vi "AIT 1553 - Write FIFOs.vi"(5 "Bus Section":T1, 7 "Mode":T2, 8 "error in (no error)":errorcluster, 11 "RT Data in":T3 {"Acyclic Frame Refs" format="%.0x"; "Label Transfer Config"."Block Data Refs"."Data Reference" format="%.0x"; "Status Config"."HWOut Dur Ref" format="%.0x"; "Status Config"."HWIn Dur Ref" format="%.0x"; "Status Config"."HWOut Count Ref" format="%.0x"; "Status Config"."HWIn Count Ref" format="%.0x"; "Status Config"."Error Data Ref" format="%.0x"; "HWOutput Channels"."Message Settings"."Driver Data"."First Word" min=8 max=31; "HWOutput Channels"."Message Settings"."Driver Data"."Num Bits" min=1 max=32; "HWOutput Channels"."Message Settings"."Driver Data"."Start Bit" min=8 max=31; "HWOutput Channels"."Message Settings"."Block Data Refs"."Data Reference" format="%.0x"; "HWInput Channels"."Message Settings"."Driver Data"."First Word" min=8 max=31; "HWInput Channels"."Message Settings"."Driver Data"."Num Bits" min=1 max=32; "HWInput Channels"."Message Settings"."Driver Data"."Start Bit" min=8 max=31; "HWInput Channels"."Message Settings"."Block Data Refs"."Data Reference" format="%.0x"}) -> (0 "error out":errorcluster, 3 "RT Data out":T3 {"Acyclic Frame Refs" format="%.0x"; "Label Transfer Config"."Block Data Refs"."Data Reference" format="%.0x"; "Status Config"."HWOut Dur Ref" format="%.0x"; "Status Config"."HWIn Dur Ref" format="%.0x"; "Status Config"."HWOut Count Ref" format="%.0x"; "Status Config"."HWIn Count Ref" format="%.0x"; "Status Config"."Error Data Ref" format="%.0x"; "HWOutput Channels"."Message Settings"."Driver Data"."First Word" min=8 max=31; "HWOutput Channels"."Message Settings"."Driver Data"."Num Bits" min=1 max=32; "HWOutput Channels"."Message Settings"."Driver Data"."Start Bit" min=8 max=31; "HWOutput Channels"."Message Settings"."Block Data Refs"."Data Reference" format="%.0x"; "HWInput Channels"."Message Settings"."Driver Data"."First Word" min=8 max=31; "HWInput Channels"."Message Settings"."Driver Data"."Num Bits" min=1 max=32; "HWInput Channels"."Message Settings"."Driver Data"."Start Bit" min=8 max=31; "HWInput Channels"."Message Settings"."Block Data Refs"."Data Reference" format="%.0x"})   [LabVIEW 2013, in "AIT 1553 Custom Device.lvlib"]
uses:
  AIT 1553 Custom Device.lvlib
  RT Controls/AIT 1553  - RT Data.ctl
  RT Controls/AIT 1553 - RT HW Channel.ctl
  RT Controls/AIT 1553 - Bus Section.ctl
  RT Controls/AIT 1553 - RT Message Settings.ctl
  <vilib>/NI Veristand/Custom Device API/Block Data Reference.ctl
  <vilib>/NI Veristand/Custom Device API/Data Reference.ctl
  RT Controls/AIT 1553 - Driver Data.ctl
  Controls and Global/Start Bit.ctl
  Controls and Global/Number of Bits.ctl
  RT Controls/AIT 1553 - Board Config Info.ctl
  RT Controls/AIT 1553 - Hardware Type.ctl
  RT Controls/Error Qs.ctl
  RT Controls/Status Channels Config.ctl
  RT Controls/FIFO.ctl
  RT Controls/Label Transfer Config.ctl
  <vilib>/NI Veristand/Custom Device API/Custom Device Item Ref.ctl
  RT Controls/ReadWrite Selector.ctl
  <vilib>/NI Veristand/Custom Device API/Custom Device API.lvlib
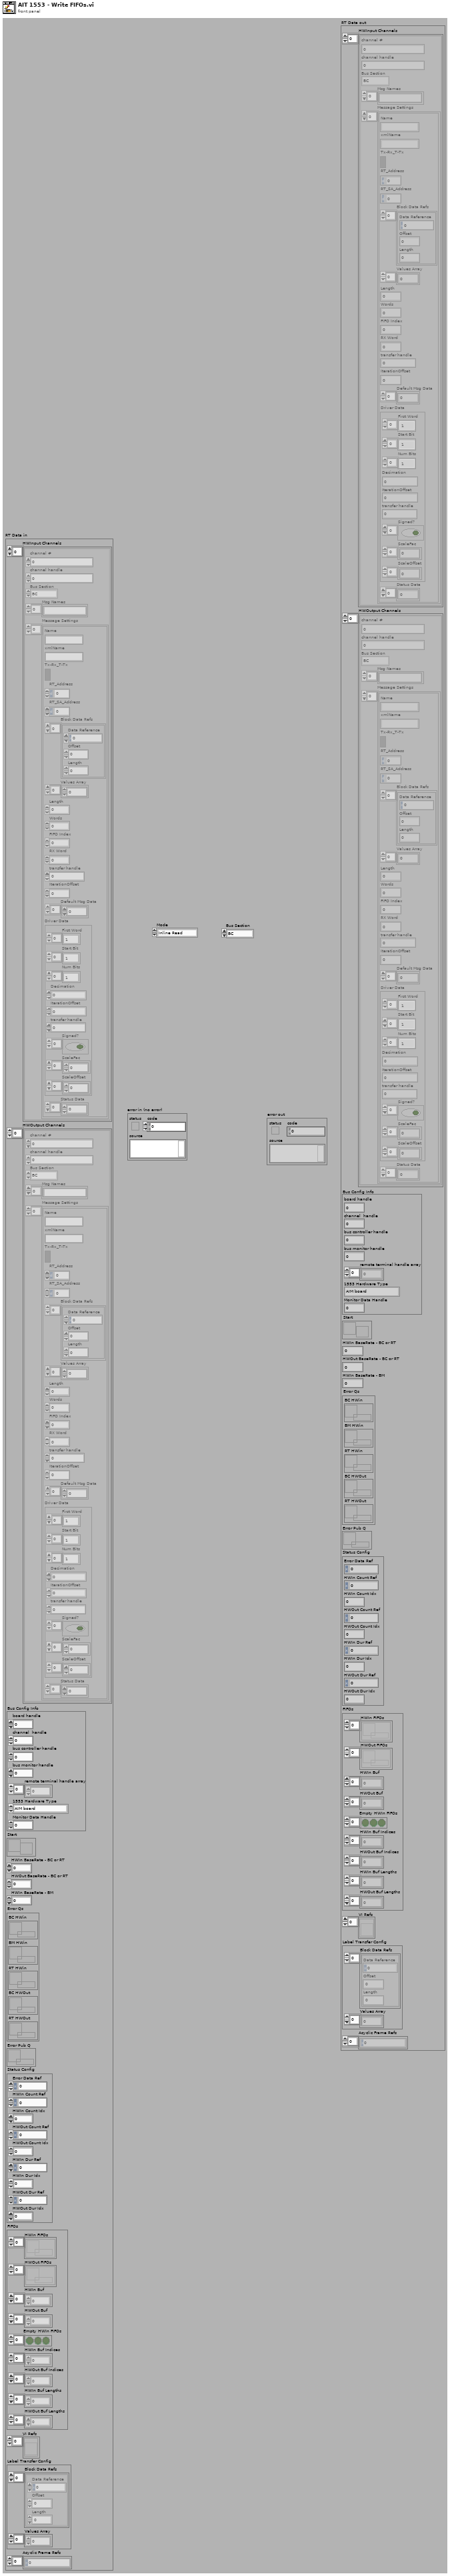
[diagram p1: front panel]
types:
  T1 = typedef "AIT 1553 Custom Device.lvlib/AIT 1553 - Bus Section.ctl" = enum16{"BC", "BM", "RT"}
  T2 = typedef "AIT 1553 Custom Device.lvlib/ReadWrite Selector.ctl" = enum16{"Inline Read", "Inline Write", "Async HWIn", "Async HWOut"}
  T3 = typedef "AIT 1553 Custom Device.lvlib/AIT 1553  - RT Data.ctl" = cluster{"HWInput Channels":T4[], "HWOutput Channels":T4[], "Bus Config Info":T11, "Start":refnum<notifier>, "HWIn BaseRate - BC or RT":i64, "HWOut BaseRate - BC or RT":i64, "HWIn BaseRate - BM":i64, "Error Qs":T13, "Error Pub Q":refnum<queue>, "Status Config":T14, "FIFOs":T15, "VI Refs":refnum<vi>[], "Label Transfer Config":T16, "Acyclic Frame Refs":T17[]}
  T4 = typedef "AIT 1553 Custom Device.lvlib/AIT 1553 - RT HW Channel.ctl" = cluster{"channel #":u16, "channel handle":u32, "Bus Section":T1, "Msg Names":string[], "Message Settings":T5[]}
  T5 = typedef "AIT 1553 Custom Device.lvlib/AIT 1553 - RT Message Settings.ctl" = cluster{"Name":string, "xmlName":string, "Tx-Rx_T-Tx":bool, "RT_Address":u8, "RT_SA_Address":u8, "Block Data Refs":T6[], "Values Array":dbl[], "Length":i32, "Words":i32, "FIFO Index":i32, "RX Word":u32, "transfer handle":u32, "IterationOffset":i32, "Default Msg Data":u16[], "Driver Data":T8, "Status Data":u32[]}
  T6 = typedef "Custom Device API.lvlib/Block Data Reference.ctl" = cluster{"Data Reference":T7, "Offset":i32, "Length":i32}
  T7 = typedef "Custom Device API.lvlib/Data Reference.ctl" = i32
  T8 = typedef "AIT 1553 Custom Device.lvlib/AIT 1553 - Driver Data.ctl" = cluster{"First Word":T9[], "Start Bit":T9[], "Num Bits":T10[], "Decimation":i32, "IterationOffset":i32, "transfer handle":u32, "Signed?":bool[], "ScaleFac":dbl[], "ScaleOffset":dbl[]}
  T9 = typedef "AIT 1553 Custom Device.lvlib/Start Bit.ctl" = i32
  T10 = typedef "AIT 1553 Custom Device.lvlib/Number of Bits.ctl" = i32
  T11 = typedef "AIT 1553 Custom Device.lvlib/AIT 1553 - Board Config Info.ctl" = cluster{"board handle":u32, "channel  handle":u32, "bus controller handle":u32, "bus monitor handle":u32, "remote terminal handle array":u32[], "1553 Hardware Type":T12, "Monitor Data Handle":u32}
  T12 = typedef "AIT 1553 Custom Device.lvlib/AIT 1553 - Hardware Type.ctl" = enum16{"AIM board", "AIT Board"}
  T13 = typedef "AIT 1553 Custom Device.lvlib/Error Qs.ctl" = cluster{"BC HWin":refnum<queue>, "BM HWin":refnum<queue>, "RT HWin":refnum<queue>, "BC HWOut":refnum<queue>, "RT HWOut":refnum<queue>}
  T14 = typedef "AIT 1553 Custom Device.lvlib/Status Channels Config.ctl" = cluster{"Error Data Ref":T7, "HWIn Count Ref":T7, "HWIn Count Idx":i32, "HWOut Count Ref":T7, "HWOut Count Idx":i32, "HWIn Dur Ref":T7, "HWIn Dur Idx":i32, "HWOut Dur Ref":T7, "HWOut Dur Idx":i32}
  T15 = typedef "AIT 1553 Custom Device.lvlib/FIFO.ctl" = cluster{"HWIn FIFOs":refnum<k33>[], "HWOut FIFOs":refnum<k33>[], "HWIn Buf":dbl[], "HWOut Buf":dbl[], "Empty HWIn FIFOs":bool[], "HWIn Buf Indices":i32[], "HWOut Buf Indices":i32[], "HWIn Buf Lengths":i32[], "HWOut Buf Lengths":i32[]}
  T16 = typedef "AIT 1553 Custom Device.lvlib/Label Transfer Config.ctl" = cluster{"Block Data Refs":T6[], "Values Array":dbl[]}
  T17 = typedef "Custom Device API.lvlib/Custom Device Item Ref.ctl" = u64
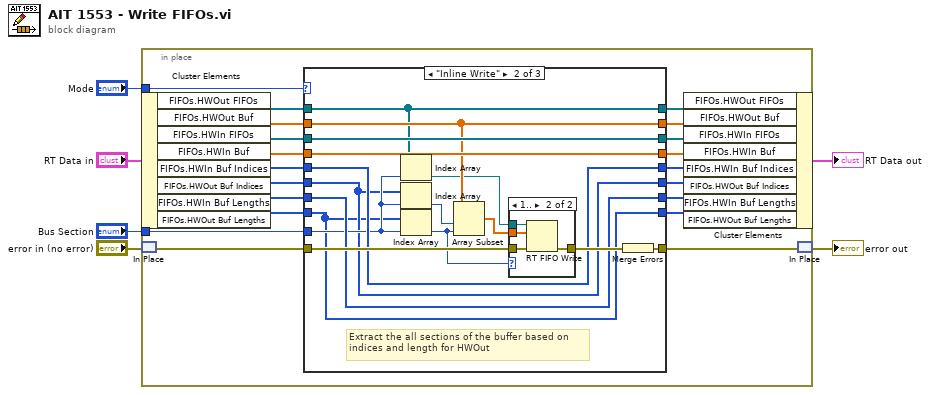
[diagram p0: block diagram]
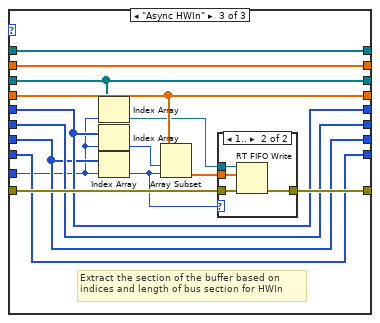
[diagram p4: hidden frame]
diagram:
  n1 = in-place {
    in-place-border: "Mode" -> [w20]
    in-place-border: "Bus Section" -> [w7]
    n2 = in-place-cluster #1("RT Data in") -> ("FIFOs.HWOut FIFOs"=w19:refnum<k33>[], "FIFOs.HWOut Buf"=w18:dbl[], "FIFOs.HWIn FIFOs"=w26:refnum<k33>[], "FIFOs.HWIn Buf"=w25:dbl[], "FIFOs.HWIn Buf Indices"=w15:i32[], "FIFOs.HWOut Buf Indices"=w14:i32[], "FIFOs.HWIn Buf Lengths"=w13:i32[], "FIFOs.HWOut Buf Lengths"=w12:i32[])
    n3 = in-place-match #2("error in (no error)") -> (w22:errorcluster)
    n4 = case shown="\"Inline Write\"" w20 {
      tunnel: w26 -> [w34 w49 w60]
      tunnel: w25 -> [w35 w50 w65]
      tunnel: [w35 w50 w65] -> w24
      tunnel: [w34 w49 w60] -> w23
      tunnel: w22 -> [w33 w51 w69]
      tunnel: [w33 w46 w68] -> w21
      tunnel: w19 -> [w31 w45 w71]
      tunnel: w18 -> [w32 w47 w70]
      tunnel: [w31 w45 w71] -> w17
      tunnel: [w32 w47 w70] -> w16
      tunnel: [w30 w43 w63] -> w11
      tunnel: w15 -> [w30 w43 w63]
      tunnel: [w29 w37 w66] -> w10
      tunnel: w14 -> [w29 w37 w66]
      tunnel: [w28 w42 w62] -> w9
      tunnel: w13 -> [w28 w42 w62]
      tunnel: [w27 w36 w67] -> w8
      tunnel: w12 -> [w27 w36 w67]
      tunnel: w7 -> [_ w41 w59]
      frame Default {
      }
      frame "Inline Write" {
        # "Extract the all sections of the buffer based on \nindices and length for HWOut"
        n5 = Index Array(array=w45, index=w41) -> (element=w44:refnum<k33>)
        n6 = Index Array(array=w37, index=w41) -> (element=w40:i32)
        n7 = Index Array(array=w36, index=w41) -> (element=w38:i32)
        n8 = Array Subset(array=w47, index=w40, length=w38) -> (w39:dbl[])
        n9 = case shown="1.." w38 {
          tunnel: w51 -> [w52 w56]
          tunnel: [w52 w55] -> w48
          tunnel: w44 -> [_ w54]
          tunnel: w39 -> [_ w53]
          frame 0, Default {
          }
          frame 1.. {
            n10 = RT FIFO Write(0:w54, 1:w53, 3:w56) -> (11:w55:errorcluster)  [unwired: 2 in, 3 out]
          }
        }
        n11 = Merge Errors(w48) -> (w46:errorcluster)
      }
      frame "Async HWIn" {
        # "Extract the section of the buffer based on \nindices and length of bus section for HWIn"
        n12 = Index Array(array=w60, index=w59) -> (element=w58:refnum<k33>)
        n13 = Index Array(array=w63, index=w59) -> (element=w61:i32)
        n14 = Index Array(array=w62, index=w59) -> (element=w57:i32)
        n15 = Array Subset(array=w65, index=w61, length=w57) -> (w64:dbl[])
        n16 = case shown="1.." w57 {
          tunnel: w69 -> [w72 w76]
          tunnel: [w72 w75] -> w68
          tunnel: w64 -> [_ w74]
          tunnel: w58 -> [_ w73]
          frame 0, Default {
          }
          frame 1.. {
            n17 = RT FIFO Write(0:w73, 1:w74, 3:w76) -> (11:w75:errorcluster)  [unwired: 2 in, 3 out]
          }
        }
      }
    }
    n18 = in-place-cluster #1("FIFOs.HWOut FIFOs"=w17, "FIFOs.HWOut Buf"=w16, "FIFOs.HWIn FIFOs"=w23, "FIFOs.HWIn Buf"=w24, "FIFOs.HWIn Buf Indices"=w11, "FIFOs.HWOut Buf Indices"=w10, "FIFOs.HWIn Buf Lengths"=w9, "FIFOs.HWOut Buf Lengths"=w8) -> (→"RT Data out":T3)
    n19 = in-place-match #2(w21) -> (→"error out":errorcluster)
  }
